vi "檢測_Line_Sub.vi"(6 "邊參數":T2={"Search Direction"=0, "Edge Polarity"=0, "Kernel Size"=3, "Width"=3, "Minimum Edge Strength"=10.0} {"Minimum Edge Strength" format="%.2f"; "Width" step=2; "Kernel Size" step=2; "Edge Polarity" items=["All Edges", "Rising Edges", "Falling Edges"]; "Search Direction" items=["Left to Right", "Right to Left", "Top to Bottom", "Bottom to Top"]}, 8 "error in (no error)":errorcluster, 9 "ROI":T6, 10 "Coordinate System":T5 {"Measurement System"."Axis Reference" items=["Direct", "Indirect"]; "Measurement System"."Angle (deg)" format="%.2f"; "Measurement System"."Origin"."Y" format="%.2f"; "Measurement System"."Origin"."X" format="%.2f"; "Reference System"."Axis Reference" items=["Direct", "Indirect"]; "Reference System"."Angle (deg)" format="%.2f"; "Reference System"."Origin"."Y" format="%.2f"; "Reference System"."Origin"."X" format="%.2f"}, 11 "Image":T4) -> (0 "error out":errorcluster, 2 "線段2端點":T1 {"點2 (Pixels)"."Y" format="%.2f"; "點2 (Pixels)"."X" format="%.2f"; "點1 (Pixels)"."Y" format="%.2f"; "點1 (Pixels)"."X" format="%.2f"}, 3 "Image Out":T4)   [LabVIEW 2015]
uses:
  <vilib>/vision/Image Controls.llb/IMAQ Image.ctl
  Setting/0.Control/Setting_Control_Line Paremeter.ctl
  <vilib>/vision/Measure.llb/Edge Polarity.ctl
  <vilib>/vision/Measure.llb/Edge Options.ctl
  <vilib>/vision/Measure.llb/Straight Edge Options.ctl
  <vilib>/vision/Measure.llb/Straight Edge Process.ctl
  <vilib>/vision/NI_Vision_Development_Module.lvlib
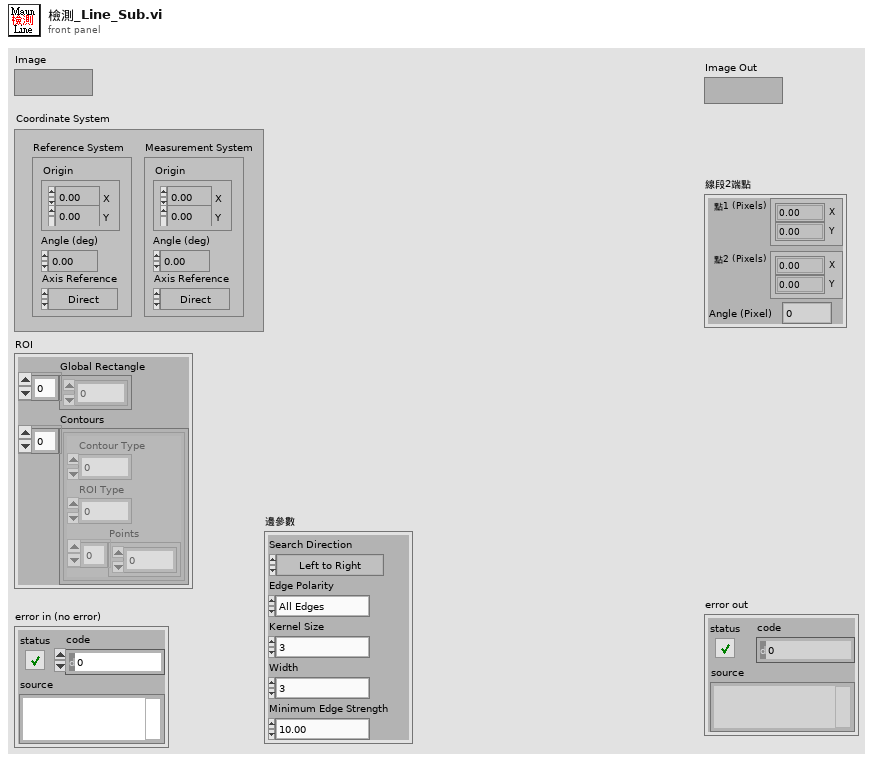
[diagram p1: front panel]
types:
  T1 = cluster{"點1 (Pixels)":cluster{"X":sgl, "Y":sgl}, "點2 (Pixels)":cluster{"X":sgl, "Y":sgl}, "Angle (Pixel)":dbl}
  T2 = typedef "Setting_Control_Line Paremeter.ctl" = cluster{"Search Direction":u32, "Edge Polarity":T3, "Kernel Size":u32, "Width":u32, "Minimum Edge Strength":sgl}
  T3 = typedef "Edge Polarity.ctl" = u32
  T4 = typedef "IMAQ Image.ctl" = refnum<image>
  T5 = typedef "IMAQ Coordinate System" = cluster{"Reference System":cluster{"Origin":cluster{"X":sgl, "Y":sgl}, "Angle (deg)":sgl, "Axis Reference":u32}, "Measurement System":cluster{"Origin":cluster{"X":sgl, "Y":sgl}, "Angle (deg)":sgl, "Axis Reference":u32}}
  T6 = cluster{"Global Rectangle":i32[], "Contours":cluster{"Contour Type":u32, "ROI Type":u32, "Points":i32[]}[]}
  T7 = typedef "Straight Edge Options.ctl" = cluster{"Number of Lines":i32, "Type":T8, "Min. Score":dbl, "Max. Score":dbl, "Orientation":dbl, "Angle Range":dbl, "Angle Tolerance":dbl, "Step Size":u32, "Min. SNR (db)":dbl, "Min. Points (%)":dbl, "Hough Iterations":i32}
  T8 = typedef "Straight Edge Process.ctl" = enum32{"First Edge Rake", "Best Edge Rake", "Hough Edge Rake", "First Edge Projection", "Best Edge Projection"}
  T9 = typedef "Edge Options.ctl" = cluster{"Edge Polarity":T3, "Kernel Size":u32, "Width":u32, "Minimum Edge Strength":sgl, "Interpolation Type":enum32{"Zero Order", "Bilinear", "Quadratic", "Cubic", "Bilinear Fixed"}, "Data Processing Method":enum32{"Average", "Median"}}
  T10 = cluster{"Search Direction":u32, "Edge Options":T9, "Show Search Area":bool, "Show Search Lines":bool, "Show Edges Found":bool, "Show Result":bool, "Search Area Color":u32, "Search Lines Color":u32, "Edge Locations Color":u32, "Result Color":u32, "Overlay Group Name":string}
  T11 = cluster{"Point1 (Pixels)":cluster{"X":sgl, "Y":sgl}, "Point2 (Pixels)":cluster{"X":sgl, "Y":sgl}, "Point1 (Real-World)":cluster{"X":sgl, "Y":sgl}, "Point2 (Real-World)":cluster{"X":sgl, "Y":sgl}, "Angle (Pixel)":dbl, "Angle (Real-World)":dbl, "Score":dbl, "Straightness":dbl, "Average SNR (db)":dbl, "Calibration Valid":bool}[]
  T12 = cluster{"Point1 (Pixels)":cluster{"X":sgl, "Y":sgl}, "Point2 (Pixels)":cluster{"X":sgl, "Y":sgl}, "Point1 (Real-World)":cluster{"X":sgl, "Y":sgl}, "Point2 (Real-World)":cluster{"X":sgl, "Y":sgl}, "Angle (Pixel)":dbl, "Angle (Real-World)":dbl, "Score":dbl, "Straightness":dbl, "Average SNR (db)":dbl, "Calibration Valid":bool}
  T13 = cluster{"Point1 (Pixels)":cluster{"X":sgl, "Y":sgl}, "Point2 (Pixels)":cluster{"X":sgl, "Y":sgl}, "Angle (Real-World)":dbl}
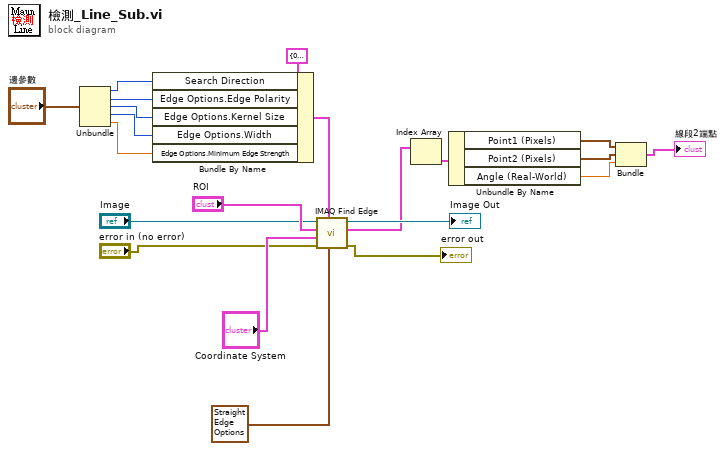
[diagram p0: block diagram]
diagram:
  n1 = Unbundle("邊參數") -> ("Search Direction"=w12:u32, "Edge Polarity"=w11:T3, "Kernel Size"=w10:u32, "Width"=w9:u32, "Minimum Edge Strength"=w8:sgl)
  n2 = Bundle By Name(cluster=T10 {"Search Direction"=0, "Edge Options"={"Edge Polarity"=0, "Kernel Size"=3, "Width"=3, "Minimum Edge Strength"=10.0, "Interpolation Type"=enum."Bilinear Fixed", "Data Processing Method"=enum."Average"}, "Show Search Area"=FALSE, "Show Search Lines"=FALSE, "Show Edges Found"=FALSE, "Show Result"=TRUE, "Search Area Color"=65280, "Search Lines Color"=255, "Edge Locations Color"=16776960, "Result Color"=16711680, "Overlay Group Name"=""} ("Options"), "Search Direction"=w12, "Edge Options.Edge Polarity"=w11, "Edge Options.Kernel Size"=w10, "Edge Options.Width"=w9, "Edge Options.Minimum Edge Strength"=w8) -> (w13:T10)
  n3 = call "IMAQ Find Edge"("Line Fit Options"=T7 {"Number of Lines"=1, "Type"=enum."First Edge Rake", "Min. Score"=10.0, "Max. Score"=1000.0, "Orientation"=0.0, "Angle Range"=45.0, "Angle Tolerance"=1.0, "Step Size"=1, "Min. SNR (db)"=0.0, "Min. Points (%)"=25.0, "Hough Iterations"=5}, "Options"=w13, "error in (no error)"="error in (no error)", "Coordinate System"="Coordinate System", "ROI Descriptor"="ROI", "Image"="Image") -> ("error out"=→"error out":errorcluster, "Straight Edges"=w7:T11, "Image Out"=→"Image Out":T4)  [unwired: 2 in, 1 out]
  n4 = Index Array(array=w7) -> (element=w6:T12)  [unwired: 1 in]
  n5 = Unbundle By Name(w6) -> ("Point1 (Pixels)"=w5:cluster{"X":sgl, "Y":sgl}, "Point2 (Pixels)"=w4:cluster{"X":sgl, "Y":sgl}, "Angle (Real-World)"=w3:dbl)
  n6 = Bundle("Point1 (Pixels)"=w5, "Point2 (Pixels)"=w4, "Angle (Real-World)"=w3) -> (→"線段2端點":T13)  [unwired: 1 in]
